vi "Read RX Data.vi"(8 "error in (no error)":errorcluster, 11 "MB_ADU_Serial in":refnum<class "MB_ADU.lvclass">) -> (0 "error out":errorcluster, 2 "RX Data":string, 3 "MB_ADU_Serial out":refnum<class "MB_ADU.lvclass">)   [LabVIEW 2023, in "Jiaxin_Stepper_Controller.lvlib" / "MB Master.lvlib" / "MB_ADU.lvclass"]
uses:
  MB_ADU.lvclass
  MB_ADU.lvclass/MB_ADU.ctl
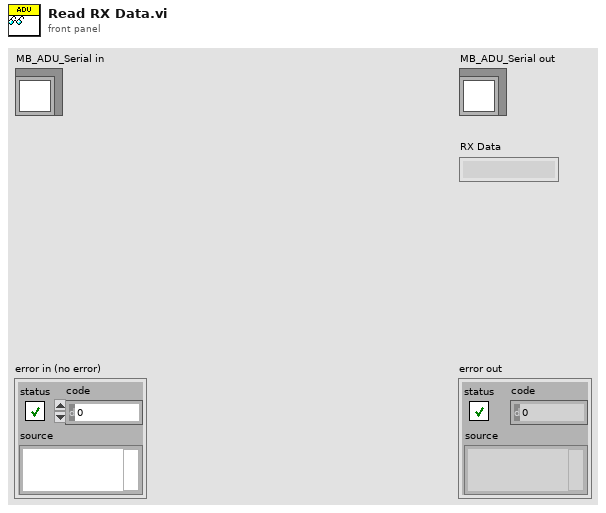
[diagram p1: front panel]
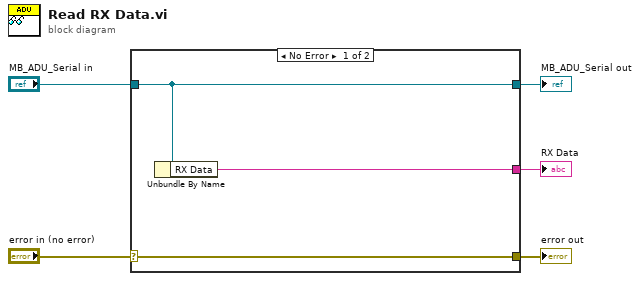
[diagram p0: block diagram]
diagram:
  n1 = case shown="No Error" "error in (no error)" {
    selector: "error in (no error)" -> [w8 w9]
    tunnel: [w8 w9] -> w4
    tunnel: [w7 w10] -> w2
    tunnel: "MB_ADU_Serial in" -> [w7 w10]
    tunnel: [w6 _] -> w1
    frame No Error {
      n2 = Unbundle By Name(w7) -> ("RX Data"=w6:string)
    }
    frame Error {
    }
  }
  "error out" <- w4
  "MB_ADU_Serial out" <- w2
  "RX Data" <- w1
